vi "FestoCPX.DO.Data.State.Set.vi"(8 "error in (no error)":errorcluster, 9 "State":bool, 10 "CPX.DO":T1) -> (0 "error out":errorcluster)   [LabVIEW 2016]
uses:
  FestoCPX.DO.Signal.ctl
  FestoCPX.DO.Data.Fglb.Action.ctl
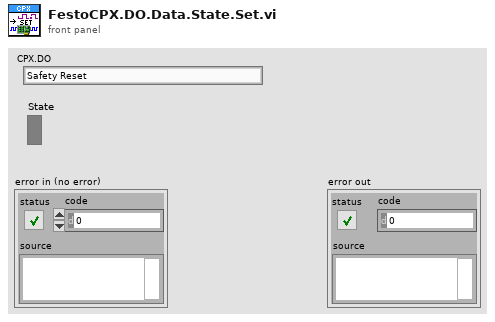
[diagram p1: front panel]
types:
  T1 = typedef "FestoCPX.DO.Signal.ctl" = enum16{"Safety Reset", "Air Main Valve", "Door Lock", "Button LED Start", "Button LED Stop", "Button LED Control", "Traffic LED Red", "Traffic LED Orange", "Traffic LED Green", "Horn", "Laser Interlock", "Laser Trigger", "Laser Fume Extractor", "Product Suction Gripper Slot 1 A", "Product Suction Gripper Slot 1 B", "Product Suction Gripper Slot 2 A", "Product Suction Gripper Slot 2 B", "Product Suction Gripper Slot 3 A", "Product Suction Gripper Slot 3 B", "Product Suction Gripper Slot 4 A", "Product Suction Gripper Slot 4 B", "Product Suction Gripper Final A", "Product Suction Gripper Final B", "Lamp", "Q1 Product Move Work", "Q1 Product Move Home", "Q2 Table Turn Work", "Q2 Table Turn Home", "Q3 Product Lift A", "Q3 Product Lift B", "Q4 Product Arm OK", "Q4 Product Arm NOK", "Q5 Product Arm Work", "Q6 Product BlowOut A", "Q6 Product BlowOut B"}
  T2 = typedef "FestoCPX.DO.Data.Fglb.Action.ctl" = enum16{"init", "set", "get", "check", "select", "reset"}
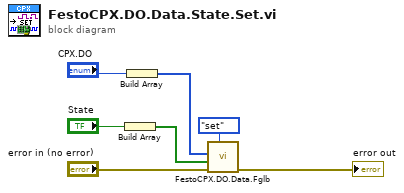
[diagram p0: block diagram]
diagram:
  n1 = Build Array("State") -> (w6:bool[])
  n2 = Build Array("CPX.DO") -> (w4:T1[])
  n3 = call "FestoCPX.DO.Data.Fglb.vi"("state (get all)"=FestoCPX.DO.Data.Fglb.Action."set", "error in (no error)"="error in (no error)", "State"=w6, "Outputs"=w4) -> ("error out"=→"error out":errorcluster)  [unwired: 5 in, 2 out]
